vi "On Launch.vi"(8 "error in (no error)":errorcluster, 11 "Hardware Resources in":T4) -> (0 "error out":errorcluster, 2 "Host Resources":T1, 3 "Hardware Resources out":T4)   [LabVIEW 2021, in "Acquisition.lvlib"]
doc: "Detect installed software and connected IO devices."
uses:
  Acquisition.lvlib
  Hardware Configuration.ctl
  Channel Settings.ctl
  IO Device.ctl
  Sensor Type.ctl
  Interval Timer/Repeat Interval.ctl
  Interval Timer/Interval Length.ctl
  Interval Timer/Interval Token.ctl
  IO API.ctl
  Host Resources.ctl
  Host Software Package.ctl
  Host IO Resource.ctl
  Interval Timer/Interval Timer.lvlib
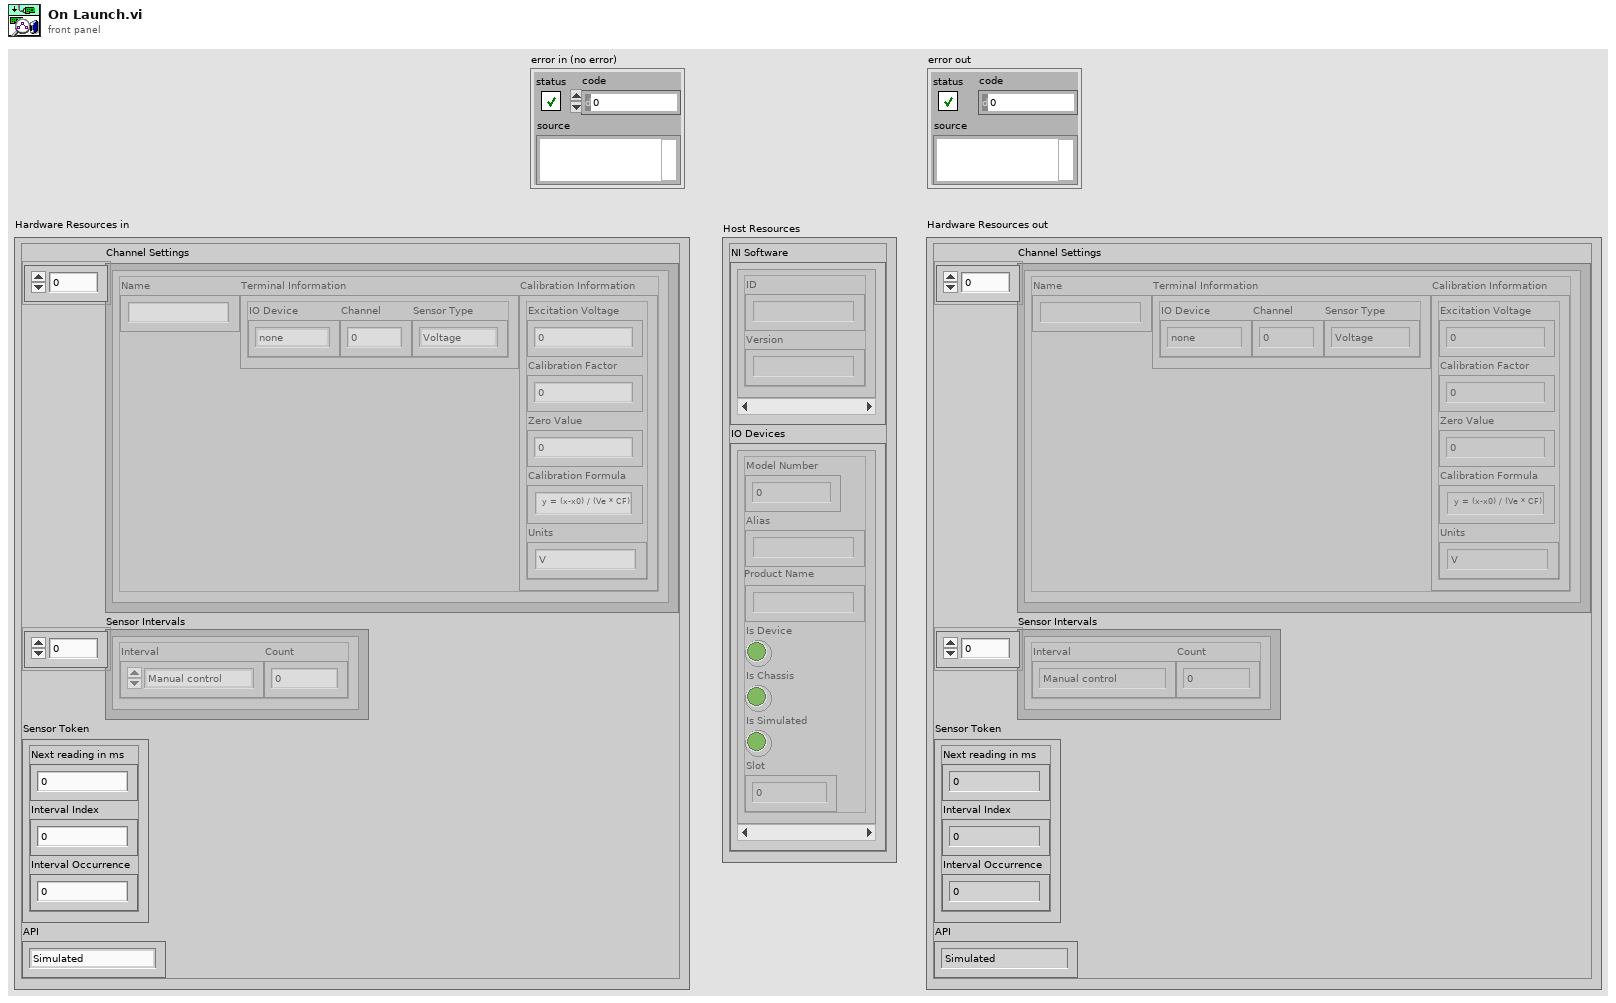
[diagram p1: front panel]
types:
  T1 = typedef "Acquisition.lvlib/Host Resources.ctl" = cluster{"NI Software":T2[], "IO Devices":T3[]}
  T2 = typedef "Acquisition.lvlib/Host Software Package.ctl" = cluster{"ID":string, "Version":string}
  T3 = typedef "Acquisition.lvlib/Host IO Resource.ctl" = cluster{"Model Number":u32, "Alias":string, "Product Name":string, "Is Device":bool, "Is Chassis":bool, "Is Simulated":bool, "Slot":i32}
  T4 = typedef "Acquisition.lvlib/Hardware Configuration.ctl" = cluster{"Channel Settings":T5[], "Sensor Intervals":T8[], "Sensor Token":T10, "API":T11}
  T5 = typedef "Acquisition.lvlib/Channel Settings.ctl" = cluster{"Name":string, "Terminal Information":cluster{"IO Device":T6, "Channel":i32, "Sensor Type":T7}, "Calibration Information":cluster{"Excitation Voltage":dbl, "Calibration Factor":dbl, "Zero Value":dbl, "Calibration Formula":string, "Units":string}}
  T6 = typedef "Acquisition.lvlib/IO Device.ctl" = enum16{"none", "9219", "9401"}
  T7 = typedef "Acquisition.lvlib/Sensor Type.ctl" = enum16{"Voltage", "Load", "Pressure", "Encoder"}
  T8 = typedef "Interval Timer.lvlib/Repeat Interval.ctl" = cluster{"Interval":T9, "Count":i32}
  T9 = typedef "Interval Timer.lvlib/Interval Length.ctl" = enum16{"Manual control", "1 second", "10 seconds", "30 seconds", "60 seconds", "600 seconds", "1200 seconds", "3600 seconds"}
  T10 = typedef "Interval Timer.lvlib/Interval Token.ctl" = cluster{"Next reading in ms":u32, "Interval Index":i32, "Interval Occurrence":i32}
  T11 = typedef "Acquisition.lvlib/IO API.ctl" = enum16{"Simulated", "DAQmx"}
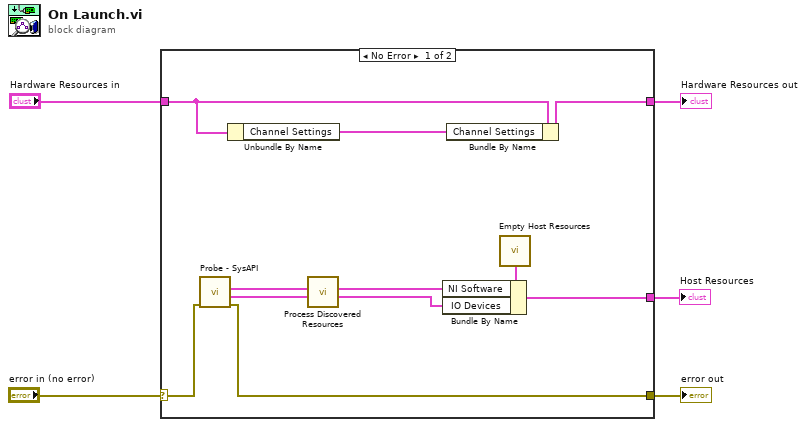
[diagram p0: block diagram]
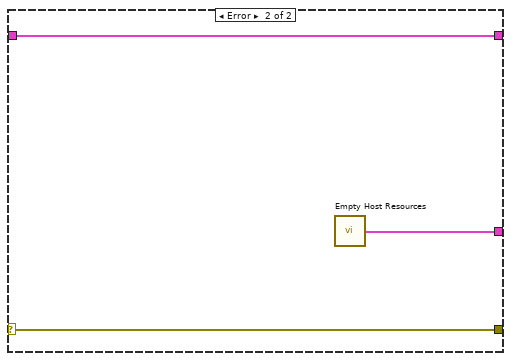
[diagram p2: hidden frame]
diagram:
  n1 = case shown="No Error" "error in (no error)" {
    selector: "error in (no error)" -> [w12 w18]
    tunnel: [w11 w18] -> w4
    tunnel: "Hardware Resources in" -> [w15 w19]
    tunnel: [w16 w19] -> w2
    tunnel: [w10 w17] -> w1
    frame No Error {
      n2 = call "Probe - SysAPI.vi"("error in (no error)"=w12) -> ("error out"=w11:errorcluster, "SysAPI Information"=w8:T3[], "NI Software Packages"=w9:T2[])  [unwired: 8 in]
      n3 = Unbundle By Name(w15) -> ("Channel Settings"=w14:T5[])
      n4 = call "Process Discovered Resources.vi"("IO Resources in"=w8, "Software Resources in"=w9) -> ("IO Resources out"=w6:T3[], "Software Resources out"=w7:T2[])  [unwired: 8 in]
      n5 = Bundle By Name(cluster=w15, "Channel Settings"=w14) -> (w16:T4)
      n6 = call "Empty Host Resources.vi"() -> ("Host Resources"=w13:T1)
      n7 = Bundle By Name(cluster=w13, "NI Software"=w7, "IO Devices"=w6) -> (w10:T1)
    }
    frame Error {
      n8 = call "Empty Host Resources.vi"() -> ("Host Resources"=w17:T1)
    }
  }
  "Hardware Resources out" <- w2
  "error out" <- w4
  "Host Resources" <- w1
